vi "Check Linear Array.vi"(8 "error in (no error)":errorcluster, 11 "Ary in":dbl[](array[numeric])=[40000000.0, 60000000.0, 80000000.0, 100000000.0, 120000000.0, 140000000.0, 160000000.0, 180000000.0, 200000000.0, 220000000.0, 240000000.0, 260000000.0, 280000000.0, 300000000.0, 320000000.0, 340000000.0, 360000000.0, 380000000.0, 400000000.0, 420000000.0, 440000000.0, 460000000.0, 480000000.0, 500000000.0, 520000000.0, 540000000.0, 560000000.0, 580000000.0, 600000000.0, 620000000.0, 640000000.0, 660000000.0, 680000000.0, 700000000.0, 720000000.0, 740000000.0, 760000000.0, 780000000.0, 800000000.0, 820000000.0, 840000000.0, 860000000.0, 880000000.0, 900000000.0, 920000000.0, 940000000.0, 960000000.0, 980000000.0, 1000000000.0, 1020000000.0, 1040000000.0, 1060000000.0, 1080000000.0, 1100000000.0, 1120000000.0, 1140000000.0, 1160000000.0, 1180000000.0, 1200000000.0, 1220000000.0, 1240000000.0, 1260000000.0, 1280000000.0, 1300000000.0, 1320000000.0, 1340000000.0, 1360000000.0, 1380000000.0, 1400000000.0, 1420000000.0, 1440000000.0, 1460000000.0, 1480000000.0, 1500000000.0, 1520000000.0, 1540000000.0, 1560000000.0, 1580000000.0, 1600000000.0, 1620000000.0, 1640000000.0, 1660000000.0, 1680000000.0, 1700000000.0, 1720000000.0, 1740000000.0, 1760000000.0, 1780000000.0, 1800000000.0, 1820000000.0, 1840000000.0, 1860000000.0, 1880000000.0, 1900000000.0, 1920000000.0, 1940000000.0, 1960000000.0, 1980000000.0, 2000000000.0, 2020000000.0, 2040000000.0, 2060000000.0, 2080000000.0, 2100000000.0, 2120000000.0, 2140000000.0, 2160000000.0, 2180000000.0, 2200000000.0, 2220000000.0, 2240000000.0, 2260000000.0, 2280000000.0, 2300000000.0, 2320000000.0, 2340000000.0, 2360000000.0, 2380000000.0, 2400000000.0, 2420000000.0, 2440000000.0, 2460000000.0, 2480000000.0, 2500000000.0, 2520000000.0, 2540000000.0, 2560000000.0, 2580000000.0, 2600000000.0, 2620000000.0, 2640000000.0, 2660000000.0, 2680000000.0, 2700000000.0, 2720000000.0, 2740000000.0, 2760000000.0, 2780000000.0, 2800000000.0, 2820000000.0, 2840000000.0, 2860000000.0, 2880000000.0, 2900000000.0, 2920000000.0, 2940000000.0, 2960000000.0, 2980000000.0, 3000000000.0]) -> (0 "error out":errorcluster, 2 "Ary size":i32=149)   [LabVIEW 2018]
doc: "This vi will check to see if an array of n elements are in linear ascending order\nAn error indicating the location of the non ascending number will be generated"
uses:
  <vilib>/Utility/error.llb/DialogType.ctl
panel:
  out "Array 2":dbl[](array[numeric])=[40000000.0, 60000000.0, 80000000.0, 100000000.0, 120000000.0, 140000000.0, 160000000.0, 180000000.0, 200000000.0, 220000000.0, 240000000.0, 260000000.0, 280000000.0, 300000000.0, 320000000.0, 340000000.0, 360000000.0, 380000000.0, 400000000.0, 420000000.0, 440000000.0, 460000000.0, 480000000.0, 500000000.0, 520000000.0, 540000000.0, 560000000.0, 580000000.0, 600000000.0, 620000000.0, 640000000.0, 660000000.0, 680000000.0, 700000000.0, 720000000.0, 740000000.0, 760000000.0, 780000000.0, 800000000.0, 820000000.0, 840000000.0, 860000000.0, 880000000.0, 900000000.0, 920000000.0, 940000000.0, 960000000.0, 980000000.0, 1000000000.0, 1020000000.0, 1040000000.0, 1060000000.0, 1080000000.0, 1100000000.0, 1120000000.0, 1140000000.0, 1160000000.0, 1180000000.0, 1200000000.0, 1220000000.0, 1240000000.0, 1260000000.0, 1280000000.0, 1300000000.0, 1320000000.0, 1340000000.0, 1360000000.0, 1380000000.0, 1400000000.0, 1420000000.0, 1440000000.0, 1460000000.0, 1480000000.0, 1500000000.0, 1520000000.0, 1540000000.0, 1560000000.0, 1580000000.0, 1600000000.0, 1620000000.0, 1640000000.0, 1660000000.0, 1680000000.0, 1700000000.0, 1720000000.0, 1740000000.0, 1760000000.0, 1780000000.0, 1800000000.0, 1820000000.0, 1840000000.0, 1860000000.0, 1880000000.0, 1900000000.0, 1920000000.0, 1940000000.0, 1960000000.0, 1980000000.0, 2000000000.0, 2020000000.0, 2040000000.0, 2060000000.0, 2080000000.0, 2100000000.0, 2120000000.0, 2140000000.0, 2160000000.0, 2180000000.0, 2200000000.0, 2220000000.0, 2240000000.0, 2260000000.0, 2280000000.0, 2300000000.0, 2320000000.0, 2340000000.0, 2360000000.0, 2380000000.0, 2400000000.0, 2420000000.0, 2440000000.0, 2460000000.0, 2480000000.0, 2500000000.0, 2520000000.0, 2540000000.0, 2560000000.0, 2580000000.0, 2600000000.0, 2620000000.0, 2640000000.0, 2660000000.0, 2680000000.0, 2700000000.0, 2720000000.0, 2740000000.0, 2760000000.0, 2780000000.0, 2800000000.0, 2820000000.0, 2840000000.0, 2860000000.0, 2880000000.0, 2900000000.0, 2920000000.0, 2940000000.0, 2960000000.0, 2980000000.0]
  out "Array":dbl[](array[numeric])=[60000000.0, 80000000.0, 100000000.0, 120000000.0, 140000000.0, 160000000.0, 180000000.0, 200000000.0, 220000000.0, 240000000.0, 260000000.0, 280000000.0, 300000000.0, 320000000.0, 340000000.0, 360000000.0, 380000000.0, 400000000.0, 420000000.0, 440000000.0, 460000000.0, 480000000.0, 500000000.0, 520000000.0, 540000000.0, 560000000.0, 580000000.0, 600000000.0, 620000000.0, 640000000.0, 660000000.0, 680000000.0, 700000000.0, 720000000.0, 740000000.0, 760000000.0, 780000000.0, 800000000.0, 820000000.0, 840000000.0, 860000000.0, 880000000.0, 900000000.0, 920000000.0, 940000000.0, 960000000.0, 980000000.0, 1000000000.0, 1020000000.0, 1040000000.0, 1060000000.0, 1080000000.0, 1100000000.0, 1120000000.0, 1140000000.0, 1160000000.0, 1180000000.0, 1200000000.0, 1220000000.0, 1240000000.0, 1260000000.0, 1280000000.0, 1300000000.0, 1320000000.0, 1340000000.0, 1360000000.0, 1380000000.0, 1400000000.0, 1420000000.0, 1440000000.0, 1460000000.0, 1480000000.0, 1500000000.0, 1520000000.0, 1540000000.0, 1560000000.0, 1580000000.0, 1600000000.0, 1620000000.0, 1640000000.0, 1660000000.0, 1680000000.0, 1700000000.0, 1720000000.0, 1740000000.0, 1760000000.0, 1780000000.0, 1800000000.0, 1820000000.0, 1840000000.0, 1860000000.0, 1880000000.0, 1900000000.0, 1920000000.0, 1940000000.0, 1960000000.0, 1980000000.0, 2000000000.0, 2020000000.0, 2040000000.0, 2060000000.0, 2080000000.0, 2100000000.0, 2120000000.0, 2140000000.0, 2160000000.0, 2180000000.0, 2200000000.0, 2220000000.0, 2240000000.0, 2260000000.0, 2280000000.0, 2300000000.0, 2320000000.0, 2340000000.0, 2360000000.0, 2380000000.0, 2400000000.0, 2420000000.0, 2440000000.0, 2460000000.0, 2480000000.0, 2500000000.0, 2520000000.0, 2540000000.0, 2560000000.0, 2580000000.0, 2600000000.0, 2620000000.0, 2640000000.0, 2660000000.0, 2680000000.0, 2700000000.0, 2720000000.0, 2740000000.0, 2760000000.0, 2780000000.0, 2800000000.0, 2820000000.0, 2840000000.0, 2860000000.0, 2880000000.0, 2900000000.0, 2920000000.0, 2940000000.0, 2960000000.0, 2980000000.0, 3000000000.0]
  # "This vi will check to see if an array of n elements are in linear ascending order\nAn error indicating the location of the non ascending number will be generated"
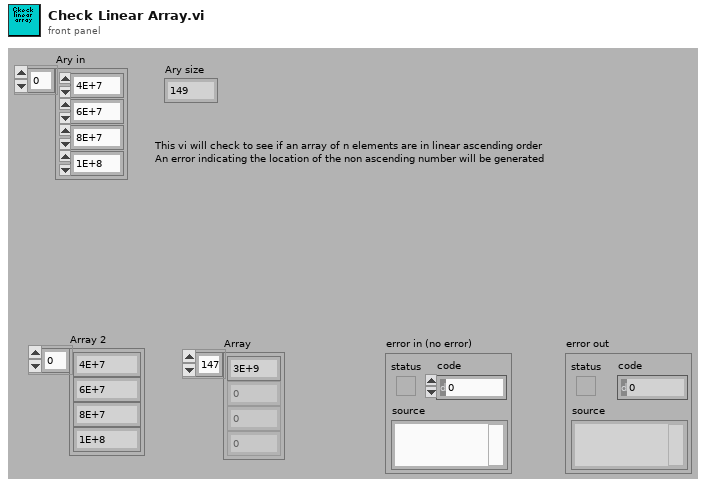
[diagram p1: front panel]
types:
  T1 = typedef "DialogType.ctl" = u16
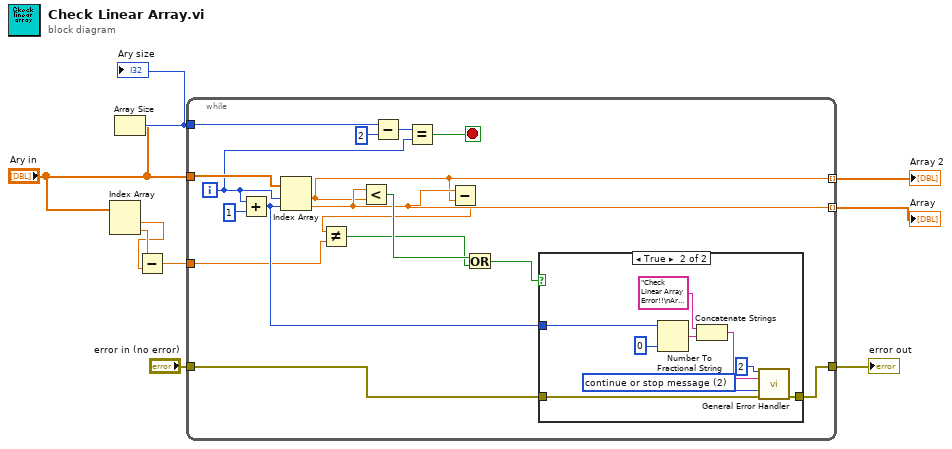
[diagram p0: block diagram]
diagram:
  n1 = Index Array(array="Ary in") -> (element #1=w2:dbl, element #2=w3:dbl)  [unwired: 2 in]
  n2 = Array Size(array="Ary in") -> (size(s)=w9:i32)
  "Ary size" <- w9
  n3 = Subtract(x=w3, y=w2) -> (x-y=w1:dbl)
  n4 = while {
    tunnel: "Ary in" -> [w26]
    tunnel: [w14] -> w8 mode=indexing
    tunnel: [w15] -> w7 mode=indexing
    tunnel: w9 -> [w23]
    tunnel: "error in (no error)" -> [w20]
    tunnel: [w19] -> w5
    tunnel: w1 -> [w12]
    i -> [w24]
    stop <- w10 stop-if-true
    n5 = Add(x=w24, y=1) -> (x+y=w17:i32)
    n6 = Index Array(array=w26, index #1=w24, index #2=w17) -> (element #1=w14:dbl, element #2=w15:dbl)
    n7 = Less?(x=w15, y=w14) -> (x < y?=w18:bool)
    n8 = Subtract(x=w23, y=2) -> (x-y=w22:i32)
    n9 = Equal?(x=w22, y=w24) -> (x = y?=w10:bool)
    n10 = Subtract(x=w15, y=w14) -> (x-y=w13:dbl)
    n11 = Not Equal?(x=w13, y=w12) -> (x != y?=w11:bool)
    n12 = Or(x=w18, y=w11) -> (x .or. y?=w16:bool)
    n13 = case shown="True" w16 {
      tunnel: [w27 w36] -> w19
      tunnel: w20 -> [w27 w34]
      tunnel: w17 -> [_ w32]
      frame False {
      }
      frame True {
        w35 = T1 2 items=["no dialog", "OK message", "continue or stop message", "OK message + warnings", "continue/stop + warnings"] ("type of dialog (OK msg:1)")
        n14 = Number To Fractional String(number=w32, precision (6)=i16 0) -> (F-format string=w30:string)  [unwired: 2 in]
        n15 = Concatenate Strings("Check Linear Array Error!!\nAry is not linear ascending...error at  line " ("[error source] (\" \")"), w30) -> (w31:string)
        n16 = call <vilib>:"General Error Handler.vi"("[error code] (0)"=2, "[error source] (\" \")"=w31, "type of dialog (OK msg:1)"=w35, "error in (no error)"=w34) -> ("error out"=w36:errorcluster)  [unwired: 7 in, 4 out]
      }
    }
  }
  "Array" <- w7
  "Array 2" <- w8
  "error out" <- w5
